vi "Example_of_single_meas_v2.vi"() -> ()   [LabVIEW 2021]
uses:
  Config_File_Paths_v2.ctl
panel:
  in  "Config files paths":T1={"ZI config file (.ini)"="Config_Ver_2\\Zurich_params.ini", "Keithley config file (.ini)"="Config_Ver_2\\Keithley_params.ini", "DAQ config file (.ini)"="Config_Ver_2\\pulse_sequence_DAQ.ini"}
  in  "Resource Address":T2={"ZI Address"="DEV714", "VISA Keithley"="KEITHLEY"}
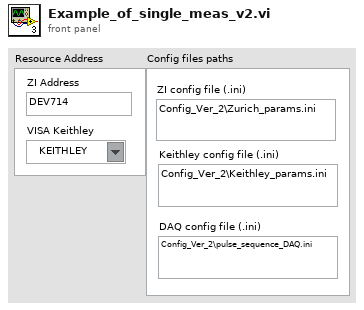
[diagram p1: front panel]
types:
  T1 = typedef "Config_File_Paths_v2.ctl" = cluster{"ZI config file (.ini)":string, "Keithley config file (.ini)":string, "DAQ config file (.ini)":string}
  T2 = cluster{"ZI Address":string, "VISA Keithley":refnum<visa-resource-name>}
  T3 = typedef "Resources_v2.ctl" = cluster{"ZI Handle":T4, "ZI ModHandle":T5, "VISA Keithley":refnum<visa-resource-name>}
  T4 = typedef "Zurich Instruments LabOne.lvlib/ziTypeHandle.ctl" = cluster{"handleValid":bool, "Conn":u64, "Path Prefix":string, "Handle":u64, "Connected":bool, "Clockbase(s)":dbl}
  T5 = typedef "Zurich Instruments LabOne.lvlib/ziTypeModHandle.ctl" = cluster{"handleValid":bool, "Conn":u64, "ModHandle":u64, "moduleID":string, "Path Prefix":string}
  T6 = typedef "ZI_Data_v2.ctl" = cluster{"R":dbl[], "Theta":dbl[], "X":dbl[], "Y":dbl[], "AuxIn0":dbl[], "AuxIn1":dbl[], "Frequency":dbl[], "DIO":dbl[], "Time":dbl[]}
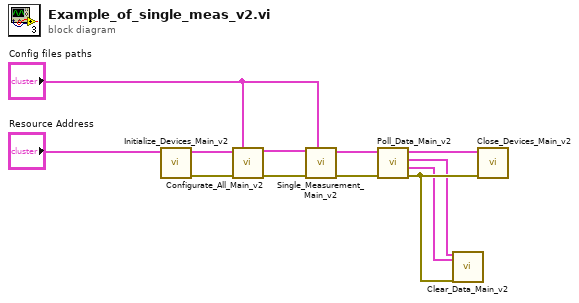
[diagram p0: block diagram]
diagram:
  n1 = call "Initialize_Devices_Main_v2.vi"("Resource Address"="Resource Address") -> ("error out"=w8:errorcluster, "Resources"=w12:T3)  [unwired: 9 in]
  n2 = call "Configurate_All_Main_v2.vi"("Resources in"=w12, "Config files paths"="Config files paths", "error in"=w8) -> ("Resources out"=w11:T3, "error out"=w7:errorcluster)  [unwired: 6 in, 5 out]
  n3 = call "Single_Measurement_Main_v2.vi"("Config files paths"="Config files paths", "error in"=w7, "Resources in"=w11) -> ("error out"=w6:errorcluster, "Resources out"=w10:T3)  [unwired: 6 in, 1 out]
  n4 = call "Poll_Data_Main_v2.vi"("error in"=w6, "Resources in"=w10) -> ("error out"=w5:errorcluster, "ZI Data 3"=w3:T6, "ZI Data 0"=w4:T6, "Resources out"=w9:T3)  [unwired: 6 in]
  n5 = call "Clear_Data_Main_v2.vi"("ZI Data 0"=w4, "ZI Data 3"=w3, "error in"=w5) -> ()  [unwired: 11 in, 6 out]
  n6 = call "Close_Devices_Main_v2.vi"("error in"=w5, "Resources"=w9) -> ()  [unwired: 9 in, 1 out]
